vi "getPLData.vi"(8 "error in (no error)":errorcluster, 10 "path":path) -> (0 "error out":errorcluster, 1 "price":dbl[][](array[numeric]), 2 "cost":dbl[][](array[numeric]), 3 "data":string[][](array[string]))   [LabVIEW 2012]
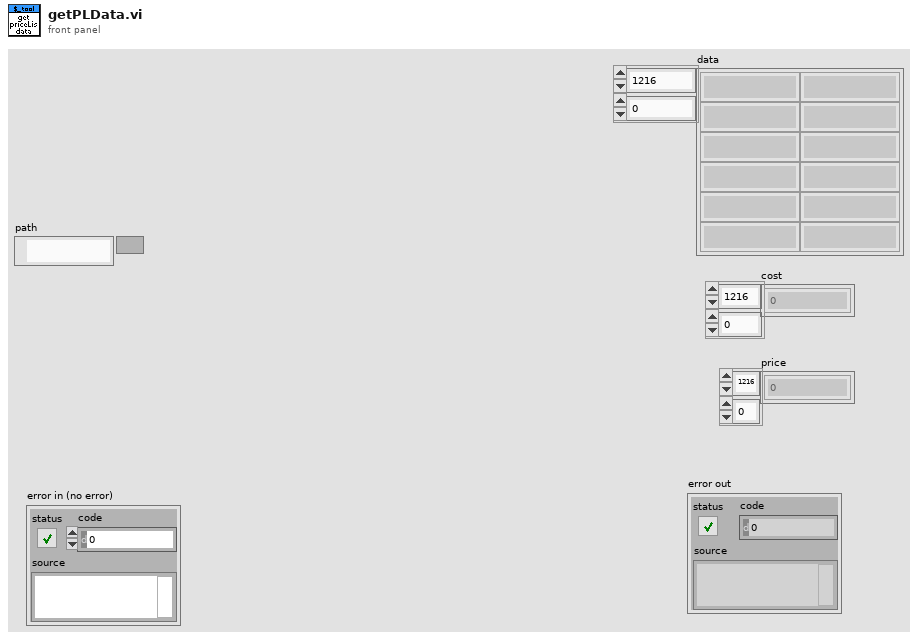
[diagram p1: front panel]
types:
  T1 = cluster{"Excel._Application":refnum<k7>, "Workbooks":refnum<k7>, "Open":refnum<k7>, "Worksheets":refnum<k7>, "Excel._Worksheet":refnum<k7>}
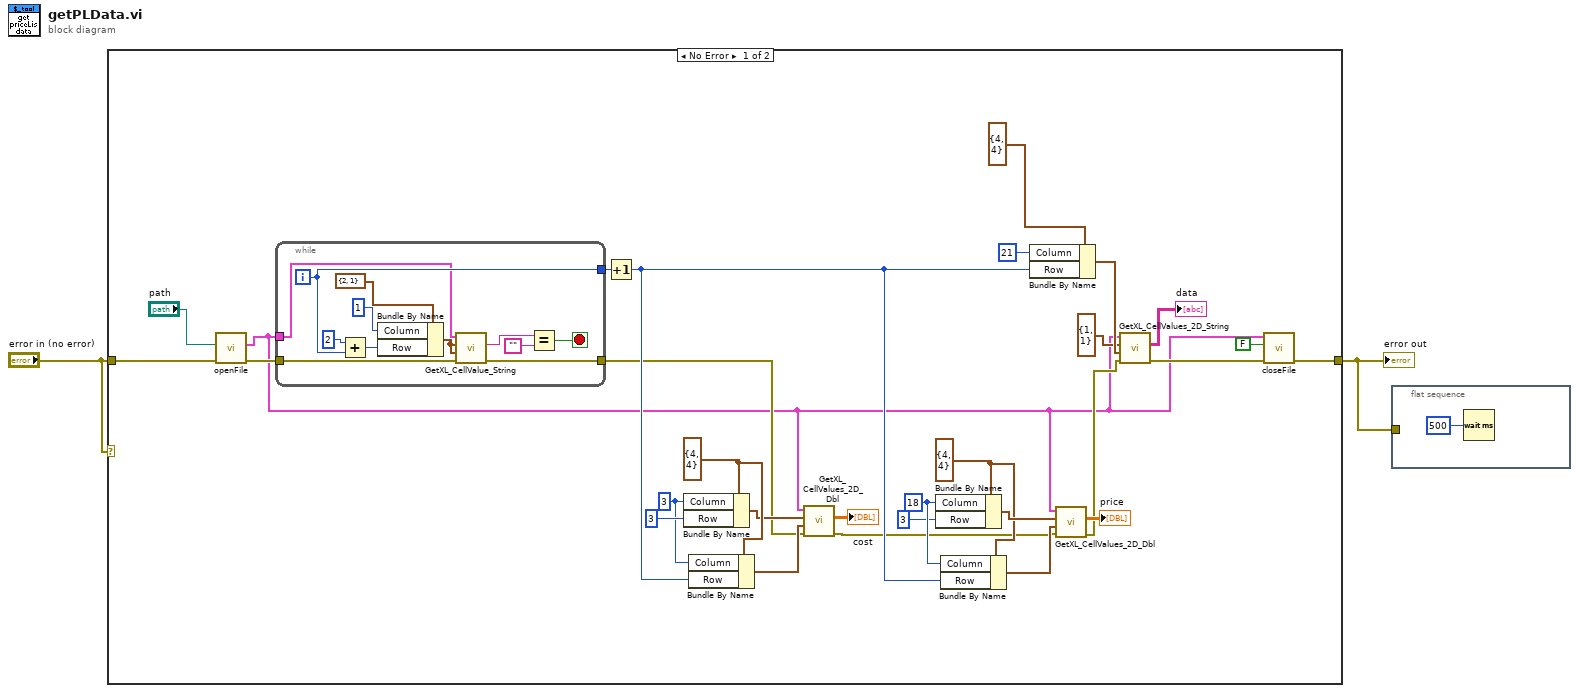
[diagram p0: block diagram]
diagram:
  n1 = case shown="No Error" "error in (no error)" {
    tunnel: "error in (no error)" -> [w9 w44]
    tunnel: [w6 w44] -> w1
    frame No Error {
      w18 = 18 ("Column")
      w14 = cluster{"Column":i32, "Row":i32} {"Column"=4, "Row"=4} ("End")
      w22 = 3 ("Column")
      w27 = cluster{"Column":i32, "Row":i32} {"Column"=4, "Row"=4} ("End")
      n2 = call "openFile.vi"("error in (no error)"=w9, "path"="path") -> ("error out"=w8:errorcluster, "Refnum Cluster Out"=w4:T1)  [unwired: 8 in]
      n3 = while {
        tunnel: w8 -> [w43]
        tunnel: [w42] -> w12
        tunnel: w4 -> [w32]
        tunnel: [w36] -> w23
        i -> [w36]
        stop <- w37 stop-if-true
        n4 = Add(x=2, y=w36) -> (x+y=w35:i32)
        n5 = Bundle By Name(cluster=cluster{"Column":i32, "Row":i32} {"Column"=2, "Row"=1} ("Start"), "Column"=1, "Row"=w35) -> (w33:cluster{"Column":i32, "Row":i32})
        n6 = call <userlib>:"GetXL_CellValue_String.vi"("error in"=w43, "End"=w33, "Start"=w33, "Refnum Cluster In"=w32) -> ("error out"=w42:errorcluster, "data"=w39:string)  [unwired: 5 in, 1 out]
        n7 = Equal?(x=w39, y="") -> (x = y?=w37:bool)
      }
      n8 = Increment(x=w23) -> (x+1=w13:i32)
      n9 = Bundle By Name(cluster=w27, "Column"=w22, "Row"=3) -> (w26:cluster{"Column":i32, "Row":i32})
      n10 = Bundle By Name(cluster=w27, "Column"=w22, "Row"=w13) -> (w25:cluster{"Column":i32, "Row":i32})
      n11 = call <userlib>:"GetXL_CellValues_2D_Dbl.vi"("error in"=w12, "End"=w25, "Start"=w26, "Refnum Cluster In"=w4) -> ("error out"=w11:errorcluster, "data"=→"cost":dbl[][])  [unwired: 5 in, 1 out]
      n12 = Bundle By Name(cluster=w14, "Column"=w18, "Row"=3) -> (w15:cluster{"Column":i32, "Row":i32})
      n13 = Bundle By Name(cluster=w14, "Column"=w18, "Row"=w13) -> (w16:cluster{"Column":i32, "Row":i32})
      n14 = Bundle By Name(cluster=cluster{"Column":i32, "Row":i32} {"Column"=4, "Row"=4} ("End"), "Column"=21, "Row"=w13) -> (w29:cluster{"Column":i32, "Row":i32})
      n15 = call <userlib>:"GetXL_CellValues_2D_Dbl.vi"("error in"=w11, "End"=w16, "Start"=w15, "Refnum Cluster In"=w4) -> ("error out"=w10:errorcluster, "data"=→"price":dbl[][])  [unwired: 5 in, 1 out]
      n16 = call <userlib>:"GetXL_CellValues_2D_String.vi"("error in"=w10, "End"=w29, "Start"=cluster{"Column":i32, "Row":i32} {"Column"=1, "Row"=1}, "Refnum Cluster In"=w4) -> ("error out"=w5:errorcluster, "data"=→"data":string[][])  [unwired: 5 in, 1 out]
      n17 = call "closeFile.vi"("error in (no error)"=w5, "Save? (F)"=FALSE, "Refnum Cluster In"=w4) -> ("error out"=w6:errorcluster)  [unwired: 8 in]
    }
    frame Error {
    }
  }
  "error out" <- w1
  n18 = flat-sequence {
    tunnel: w1 -> [_]
    frame #0 {
      n19 = Wait (ms)(milliseconds to wait=u32 500) -> ()  [unwired: 1 out]
    }
  }
